vi "GetObjectData.vi"(0 "remote ref":refnum<class "G#Object.lvclass">, 5 "error in (no error)":errorcluster) -> (13 "AppRefnum":refnum<vi>, 14 "G#DebugServer reference out":refnum<class "G#DebugServer.lvclass">, 16 "ObjectID":u32, 17 "FullClassName":string, 19 "error out":errorcluster)   [LabVIEW 2017, in "G#DebugServer.lvclass"]
doc: "Returns information about the passed object."
uses:
  <vilib>/addons/_AddQ/G#DebugServer/G#DebugServer.lvclass
  <vilib>/addons/_AddQ/G#Object/G#Object.lvclass
  <vilib>/addons/_AddQ/G#DebugServer/G#DebugServer.lvclass/G#DebugServer.ctl
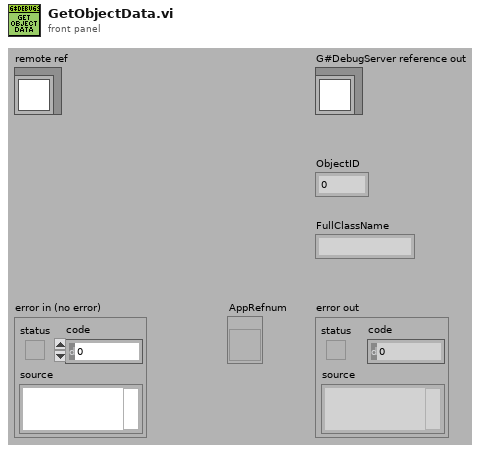
[diagram p1: front panel]
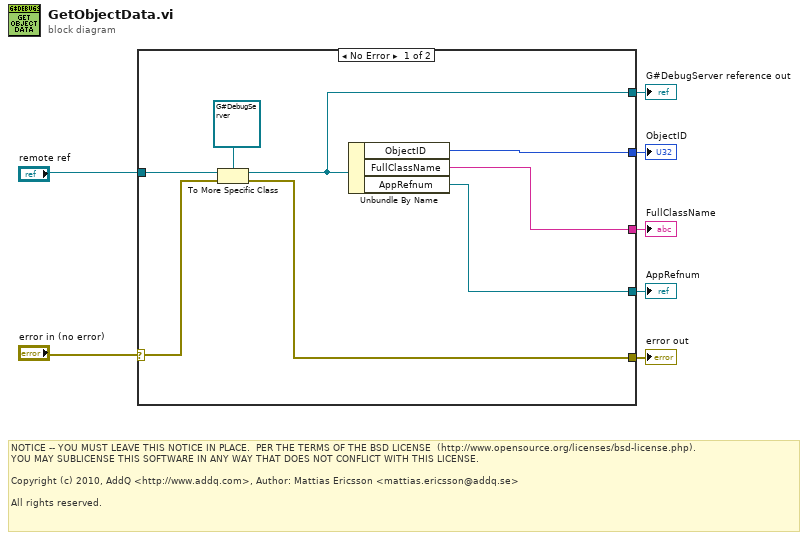
[diagram p0: block diagram]
diagram:
  # "NOTICE -- YOU MUST LEAVE THIS NOTICE IN PLACE.  PER THE TERMS OF THE BSD LICENSE  (http://www.opensource.org/licenses/bsd-license.php).\nYOU MAY SUBLICENSE THIS SOFTWARE IN ANY WAY THAT DOES NOT CONFLICT WITH THIS LICENSE.\n\nCopyright (c) 2010, AddQ <http://www.addq.com>, Author: Mattias Ericsson <mattias.ericsson@addq.se>\n\nAll rights reserved."
  n1 = case shown="No Error" "error in (no error)" {
    selector: "error in (no error)" -> [w9 w16]
    tunnel: [w15 _] -> w7
    tunnel: [w14 _] -> w6
    tunnel: [w13 _] -> w5
    tunnel: "remote ref" -> [w12 _]
    tunnel: [w10 w16] -> w3
    tunnel: [w8 _] -> w1
    frame No Error {
      n2 = To More Specific Class(target class=refnum<class "G#DebugServer.lvclass"> refnum ("G#DebugServer.lvclass"), reference=w12, error in=w9) -> (specific class reference=w8:refnum<class "G#DebugServer.lvclass">, error out=w10:errorcluster)
      n3 = Unbundle By Name(w8) -> ("ObjectID"=w15:u32, "FullClassName"=w14:string, "AppRefnum"=w13:refnum<vi>)
    }
    frame Error {
    }
  }
  "ObjectID" <- w7
  "FullClassName" <- w6
  "AppRefnum" <- w5
  "error out" <- w3
  "G#DebugServer reference out" <- w1
